vi "new_creat_control.vi"(9 "Table":string[][](table)) -> (1 "Array":T2(array[cluster]) {"Terminal Configuration" items=["default"=-1, "RSE"=10083, "NRSE"=10078, "Differential"=10106, "Pseudodifferential"=12529]})   [LabVIEW 2024]
panel:
  out "当前通道":i32
  in  "Physical Channel":tag="Dev1/ai0"
  in  "Cluster":T1={"Terminal Configuration"=-1, "Min Voltage"=-5.0, "Physical Channel"="Dev1/ai0", "Max Voltage"=5.0, "function"="", "on/off"=FALSE, "物理量"="", "单位"=""} {"Terminal Configuration" items=["default"=-1, "RSE"=10083, "NRSE"=10078, "Differential"=10106, "Pseudodifferential"=12529]}
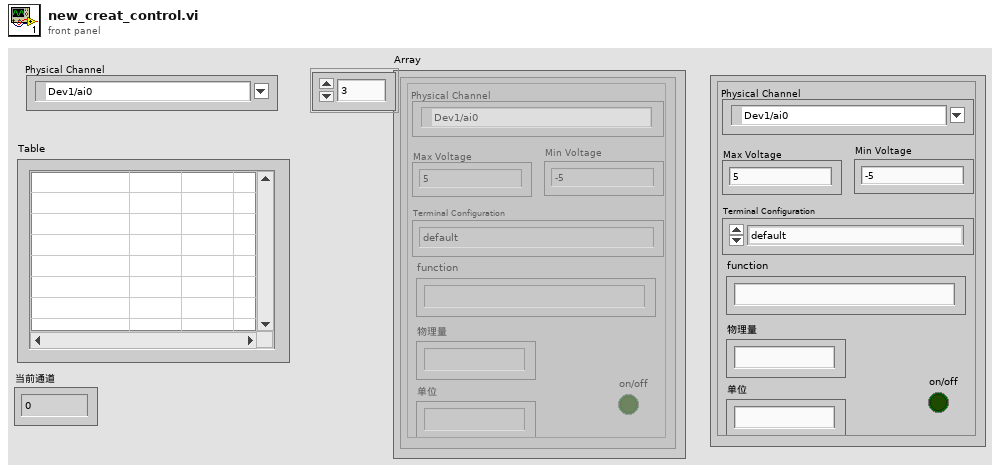
[diagram p1: front panel]
types:
  T1 = cluster{"Terminal Configuration":i32, "Min Voltage":dbl, "Physical Channel":tag, "Max Voltage":dbl, "function":string, "on/off":bool, "物理量":string, "单位":string}
  T2 = cluster{"Terminal Configuration":i32, "Min Voltage":dbl, "Physical Channel":tag, "Max Voltage":dbl, "function":string, "on/off":bool, "物理量":string, "单位":string}[]
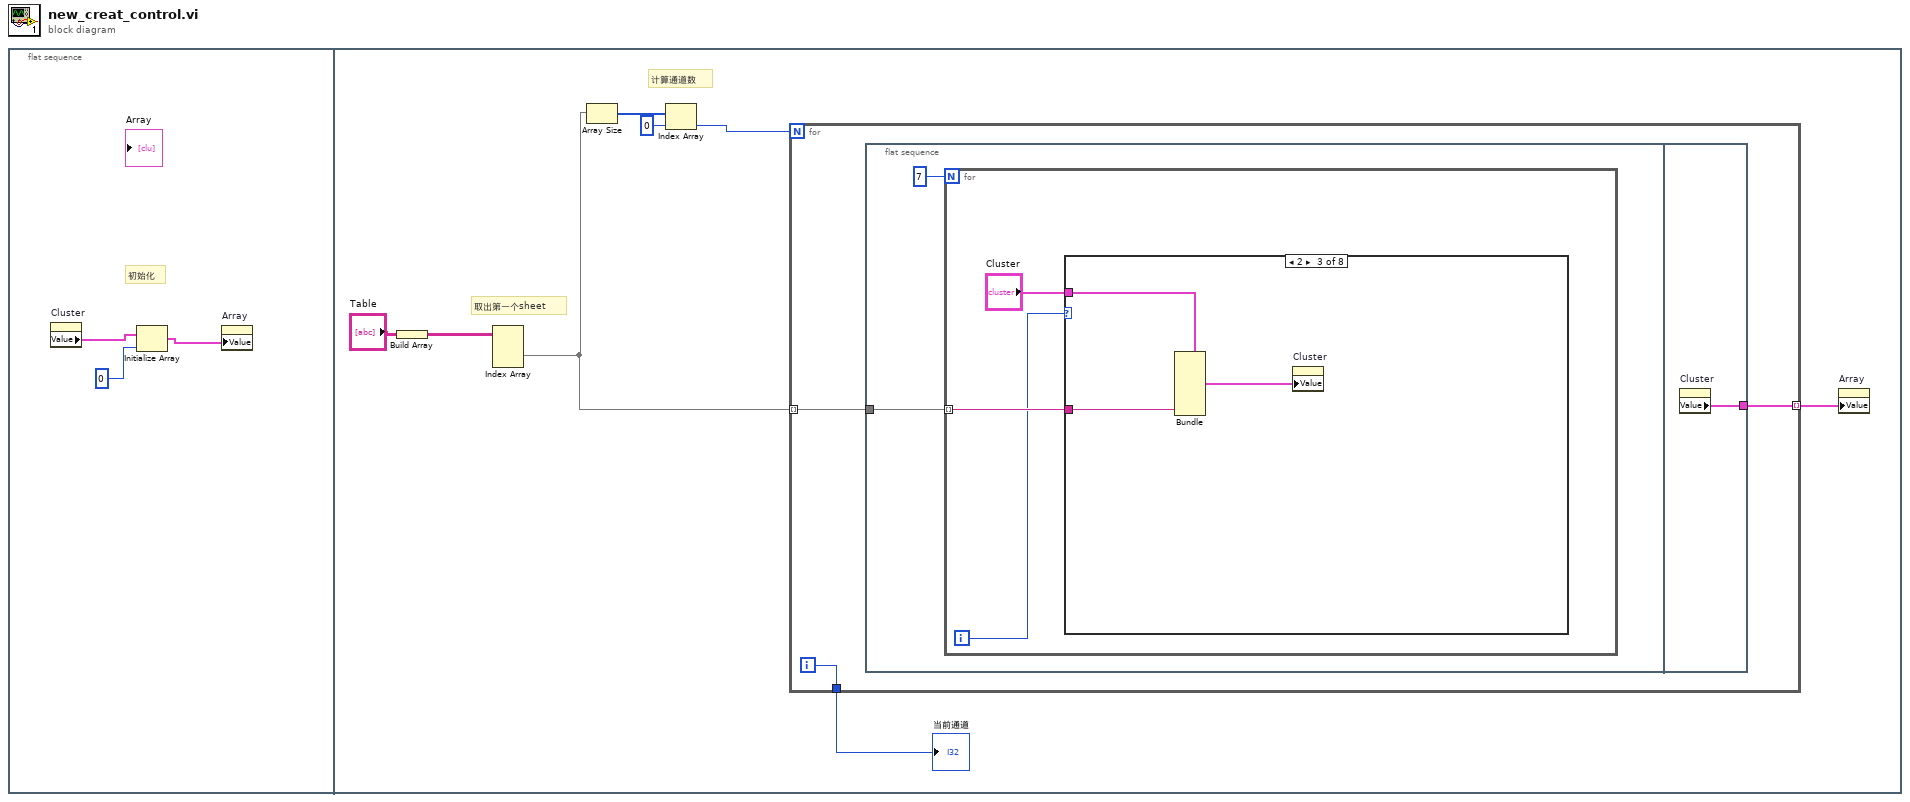
[diagram p0: block diagram]
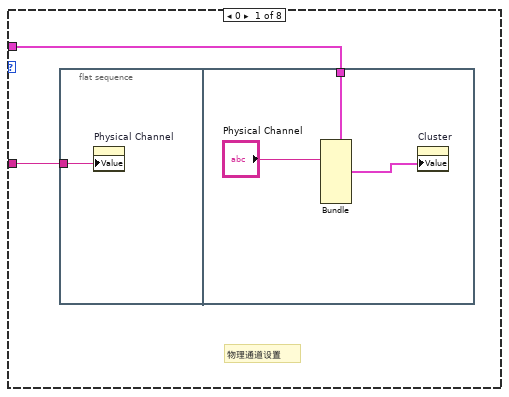
[diagram p2: hidden frame]
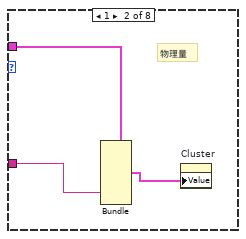
[diagram p3: hidden frame]
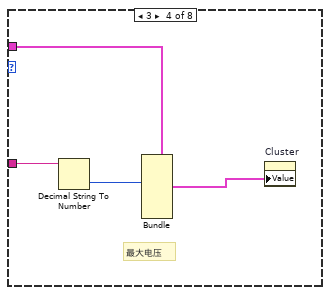
[diagram p4: hidden frame]
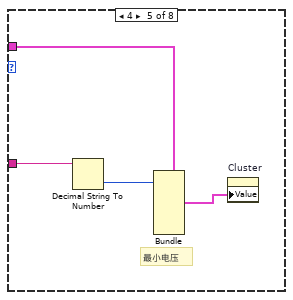
[diagram p5: hidden frame]
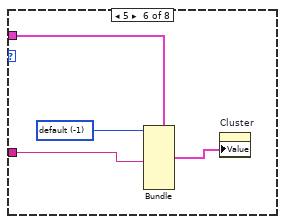
[diagram p6: hidden frame]
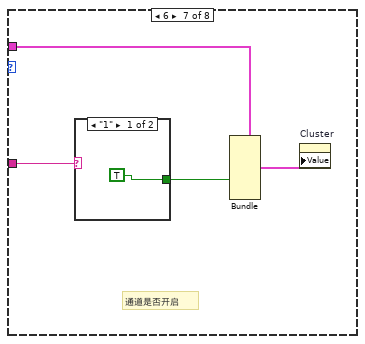
[diagram p7: hidden frame]
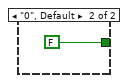
[diagram p8: hidden frame]
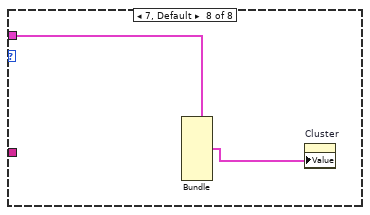
[diagram p9: hidden frame]
diagram:
  n1 = flat-sequence {
    frame #0 {
      # "初始化"
      n2 = property on="Cluster" class="Clust (strict)"() -> ("Value"=w3:T1)  [unwired: 2 in, 2 out]
      n3 = Initialize Array(w3, 0 ("dimension size")) -> (w1:T2)
      n4 = property on="Array" class="Arr (strict)"("Value"=w1) -> ()  [unwired: 2 in, 2 out]
    }
    frame #1 {
      # "计算通道数"
      # "取出第一个sheet"
      n5 = Build Array("Table") -> (w10:string[][][])
      n6 = Index Array(array=w10) -> (element=w5:string[][])  [unwired: 3 in]
      n7 = Array Size(array=w5) -> (size(s)=w9:i32[])
      n8 = Index Array(array=w9, index=0) -> (element=w4:i32)
      n9 = for {
        N: w4 -> [_]
        tunnel: w5 -> [w14] mode=indexing
        tunnel: [w13] -> w7
        tunnel: [w12] -> w6 mode=indexing
        i -> [w13]
        n10 = flat-sequence {
          tunnel: w14 -> [w15]
          tunnel: [w52] -> w12
          frame #0 {
            n11 = for {
              N: 7 -> [_]
              tunnel: w15 -> [w19] mode=indexing
              i -> [w17]
              n12 = case shown="2" w17 {
                tunnel: w19 -> [w21 w27 w30 w34 w38 w40 w45 _]
                tunnel: "Cluster" -> [w20 w28 w31 w33 w37 w42 w46 w51]
                frame 0 {
                  # "物理通道设置"
                  n13 = flat-sequence {
                    tunnel: w21 -> [w22]
                    tunnel: w20 -> [w24]
                    frame #0 {
                      n14 = property on="Physical Channel" class="DAQmxName"("Value"=w22) -> ()  [unwired: 2 in, 2 out]
                    }
                    frame #1 {
                      n15 = Bundle(cluster=w24, "Physical Channel"="Physical Channel") -> (w23:T1)  [unwired: 7 in]
                      n16 = property on="Cluster" class="Clust (strict)"("Value"=w23) -> ()  [unwired: 2 in, 2 out]
                    }
                  }
                }
                frame 1 {
                  # "物理量"
                  n17 = Bundle(cluster=w28, "物理量"=w27) -> (w26:T1)  [unwired: 7 in]
                  n18 = property on="Cluster" class="Clust (strict)"("Value"=w26) -> ()  [unwired: 2 in, 2 out]
                }
                frame 2 {
                  n19 = Bundle(cluster=w31, "单位"=w30) -> (w29:T1)  [unwired: 7 in]
                  n20 = property on="Cluster" class="Clust (strict)"("Value"=w29) -> ()  [unwired: 2 in, 2 out]
                }
                frame 3 {
                  # "最大电压"
                  n21 = Decimal String To Number(string=w34) -> (number=w35:i32)  [unwired: 2 in, 1 out]
                  n22 = Bundle(cluster=w33, "Max Voltage"=w35) -> (w32:T1)  [unwired: 7 in]
                  n23 = property on="Cluster" class="Clust (strict)"("Value"=w32) -> ()  [unwired: 2 in, 2 out]
                }
                frame 4 {
                  # "最小电压"
                  n24 = Decimal String To Number(string=w38) -> (number=w39:i32)  [unwired: 2 in, 1 out]
                  n25 = Bundle(cluster=w37, "Min Voltage"=w39) -> (w36:T1)  [unwired: 7 in]
                  n26 = property on="Cluster" class="Clust (strict)"("Value"=w36) -> ()  [unwired: 2 in, 2 out]
                }
                frame 5 {
                  w43 = -1 items=["default"=-1, "RSE"=10083, "NRSE"=10078, "Differential"=10106, "Pseudodifferential"=12529] ("Terminal Configuration")
                  n27 = Bundle(cluster=w42, "Terminal Configuration"=w43, "function"=w40) -> (w41:T1)  [unwired: 6 in]
                  n28 = property on="Cluster" class="Clust (strict)"("Value"=w41) -> ()  [unwired: 2 in, 2 out]
                }
                frame 6 {
                  # "通道是否开启"
                  n29 = case shown="\"1\"" w45 {
                    tunnel: [TRUE FALSE] -> w47
                    frame "1" {
                    }
                    frame "0", Default {
                    }
                  }
                  n30 = Bundle(cluster=w46, "on/off"=w47) -> (w44:T1)  [unwired: 7 in]
                  n31 = property on="Cluster" class="Clust (strict)"("Value"=w44) -> ()  [unwired: 2 in, 2 out]
                }
                frame 7, Default {
                  n32 = Bundle(cluster=w51) -> (w50:T1)  [unwired: 8 in]
                  n33 = property on="Cluster" class="Clust (strict)"("Value"=w50) -> ()  [unwired: 2 in, 2 out]
                }
              }
            }
          }
          frame #1 {
            n34 = property on="Cluster" class="Clust (strict)"() -> ("Value"=w52:T1)  [unwired: 2 in, 2 out]
          }
        }
      }
      "当前通道" <- w7
      n35 = property on="Array" class="Arr (strict)"("Value"=w6) -> ()  [unwired: 2 in, 2 out]
    }
  }
